vi "tbh.vi"(1 "Gain":dbl=0.001, 2 "Act":dbl, 3 "Cmd":dbl) -> (0 "Out":dbl)   [LabVIEW 2012]
panel:
  out "Error":dbl=-485.8692080184028
  out "H0":dbl=-30.366825501150174
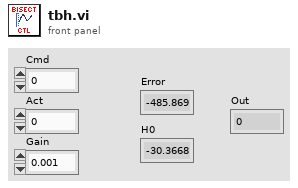
[diagram p1: front panel]
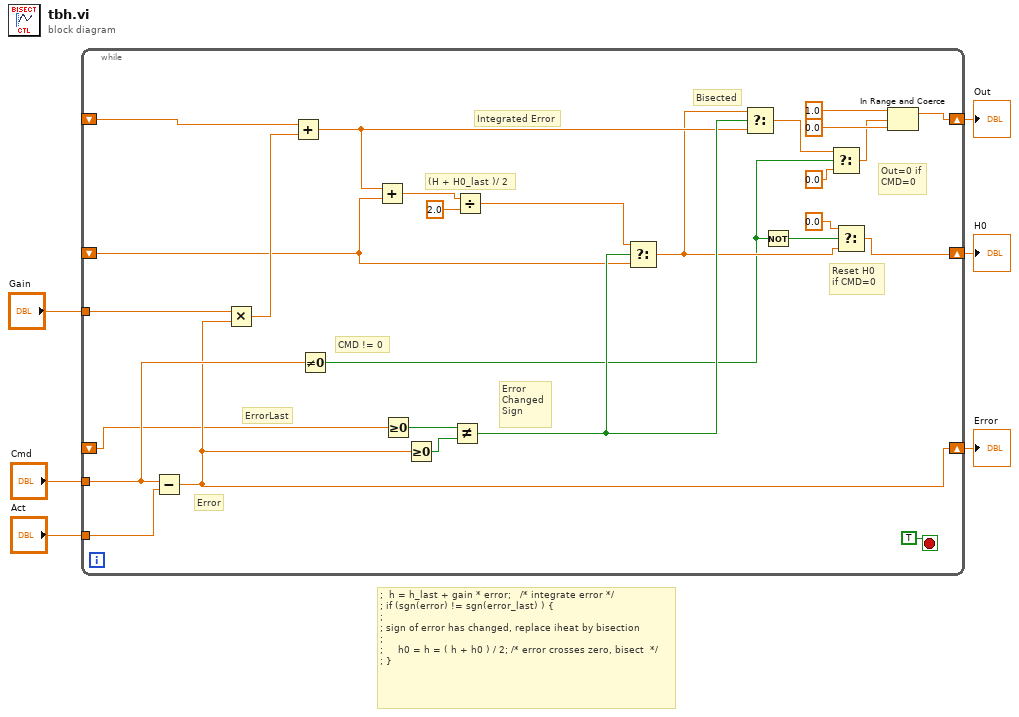
[diagram p0: block diagram]
diagram:
  # "; \th = h_last + gain * error;\t\t\t/* integrate error */\n;\tif (sgn(error) != sgn(error_last) ) {\n;\n; sign of error has changed, replace iheat by bisection\n;\n;\t    h0 = h = ( h + h0 ) / 2;\t/* error crosses zero, bisect  */\n;\t}"
  n1 = while {
    shift-right: [w14] -> w2
    shift-left: _ -> [w26]
    tunnel: "Cmd" -> [w16]
    tunnel: "Act" -> [w32]
    shift-right: [w9] -> w1
    shift-left: _ -> [w8]
    shift-right: [w20] -> w3
    shift-left: _ -> [w30]
    tunnel: "Gain" -> [w29]
    stop <- TRUE stop-if-true
    # "CMD != 0"
    # "Out=0 if\nCMD=0"
    # "Reset H0\nif CMD=0"
    # "ErrorLast"
    # "Bisected"
    # "Integrated Error"
    # "(H + H0_last )/ 2"
    # "Error\nChanged\nSign"
    # "Error"
    n2 = Subtract(x=w16, y=w32) -> (x-y=w9:dbl)
    n3 = Multiply(x=w29, y=w9) -> (x*y=w28:dbl)
    n4 = Add(x=w30, y=w28) -> (x+y=w27:dbl)
    n5 = Not Equal To 0?(x=w16) -> (x != 0?=w13:bool)
    n6 = Add(x=w27, y=w26) -> (x+y=w25:dbl)
    n7 = Greater Or Equal To 0?(x=w8) -> (x >= 0?=w7:bool)
    n8 = Greater Or Equal To 0?(x=w9) -> (x >= 0?=w10:bool)
    n9 = Not Equal?(x=w7, y=w10) -> (x != y?=w31:bool)
    n10 = Divide(x=w25, y=2.0) -> (x/y=w23:dbl)
    n11 = Select(t=w23, s=w31, f=w26) -> (s? t:f=w15:dbl)
    n12 = Select(t=w15, s=w31, f=w27) -> (s? t:f=w19:dbl)
    n13 = Not(x=w13) -> (.not. x?=w12:bool)
    n14 = Select(t=w19, s=w13, f=0.0) -> (s? t:f=w18:dbl)
    n15 = Select(t=0.0, s=w12, f=w15) -> (s? t:f=w14:dbl)
    n16 = In Range and Coerce(upper limit=1.0, x=w18, lower limit=0.0) -> (coerced(x)=w20:dbl)  [unwired: 1 out]
  }
  "Out" <- w3
  "H0" <- w2
  "Error" <- w1
